vi "Eagle_RT Send Command To GUI.vi"(8 "Error in":errorcluster, 9 "Data":variant, 11 "CMD":T1) -> (0 "error out":errorcluster)   [LabVIEW 2015]
uses:
  Stream/Controls/RT Streamer State.ctl
  Stream/Controls/RT Streamer Queue element.ctl
  Stream/LP Globals.vi
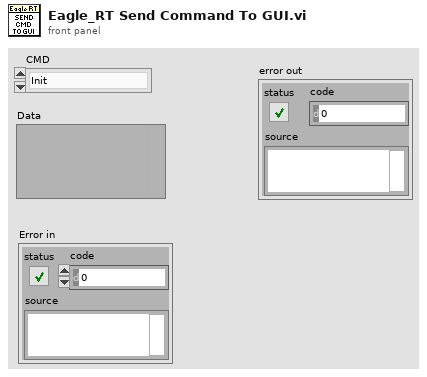
[diagram p1: front panel]
types:
  T1 = typedef "RT Streamer State.ctl" = enum16{"Init", "Idle", "Stream", "Listen", "SetRefrashRate", "SendCmdAck", "SendCmdDone", "SendSysState", "StartRecord", "Green Cordinates", "Error"}
  T2 = typedef "RT Streamer Queue element.ctl" = cluster{"CMD":T1, "Data":variant, "Error in":errorcluster}
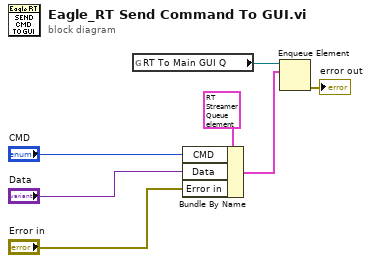
[diagram p0: block diagram]
diagram:
  n1 = global read "LP Globals.vi" "RT To Main GUI Q"() -> (w7:refnum<queue>)
  n2 = Bundle By Name(cluster=T2 {"CMD"=enum."Init", "Data"=variant, "Error in"={"status"=FALSE, "code"=0, "source"=""}} ("element"), "CMD"="CMD", "Data"="Data", "Error in"="Error in") -> (w5:T2)
  n3 = Enqueue Element(queue=w7, element=w5) -> (error out=→"error out":errorcluster)  [unwired: 2 in, 2 out]
